vi "Initialize.vi"(7 "Serial Configuration":T1={"Baud Rate"=9600, "Parity"=0, "Data Bits"=8, "Stop Bits"=10, "Flow Control"=0} {"Flow Control" items=["None", "XON/XOFF", "RTS/CTS", "XON/XOFF & RTS/CTS", "DTR/DSR", "XON/XOFF & DTR/DSR"]; "Stop Bits" items=["1.0"=10, "1.5"=15, "2.0"=20]; "Data Bits" items=["7"=7, "8"=8]; "Parity" items=["None", "Odd", "Even", "Mark", "Space"]; "Baud Rate" items=["300"=300, "600"=600, "1200"=1200, "2400"=2400, "4800"=4800, "9600"=9600, "19200"=19200]}, 8 "error in (no error)":errorcluster, 11 "VISA resource name":refnum<visa-resource-name>) -> (0 "error out":errorcluster, 3 "VISA resource name out":refnum<visa-resource-name>)   [LabVIEW 2012, in "SRS_DG535_Lib.lvlib"]
doc: "Establishes communication with the instrument and optionally performs an instrument identification query and/or an instrument reset. It also places the instrument in a default state needed for other instrument driver operations. Therefore, call this VI before calling other instrument driver VIs for this instrument. Generally, you need to call the Initialize VI only once at the beginning of an application."
uses:
  SRS_DG535_Lib.lvlib
panel:
  # "(c) 2007 <Enter Company Name Here>.  ALL RIGHTS RESERVED."
  # "EDIT: Change control description to remove example text for buses not supported."
  # "EDIT: Serial settings must match those on the physical instrument.  Review user's manual to determine the correct Flow Control protocol for the instrument.  \"None\" is the least robust option for this setting, and could lead to unreliable data transmission."
  # "EDIT: If your instrument does not support ID query or Reset, remove the ID Query or Reset control from the front panel and delete the case structure with the ID Query or Reset code from the block diagram."
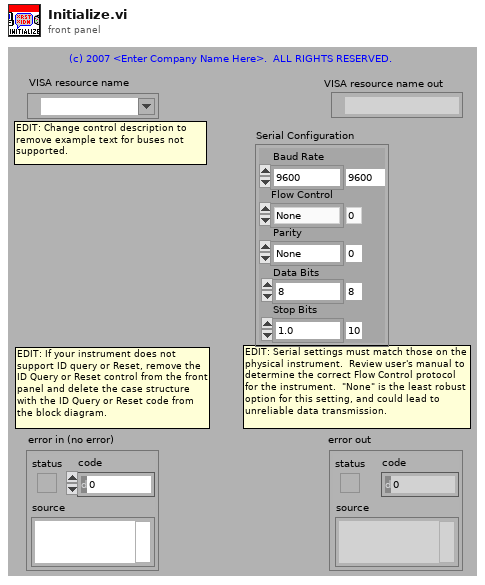
[diagram p1: front panel]
types:
  T1 = cluster{"Baud Rate":u32, "Parity":u16, "Data Bits":u16, "Stop Bits":u16, "Flow Control":u16}
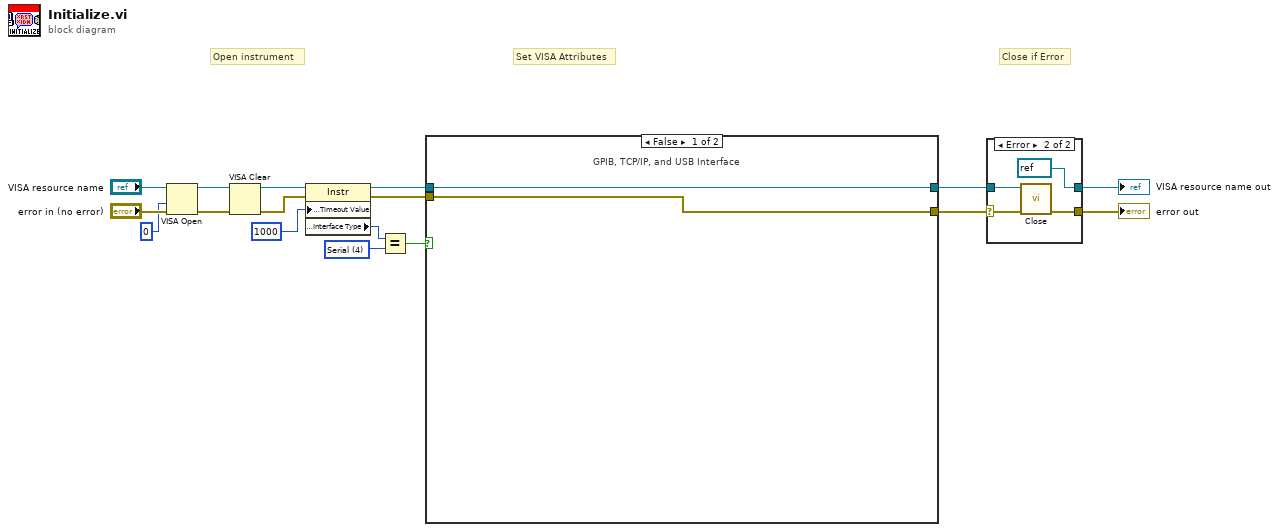
[diagram p0: block diagram]
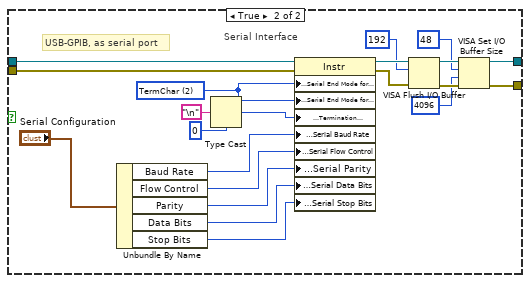
[diagram p2: hidden frame]
diagram:
  w10 = u16 4 items=["GPIB"=1, "VXI"=2, "GPIB-VXI"=3, "Serial"=4, "PXI"=5, "TCPIP"=6, "USB"=7] ("Interface Information:Interface Type")
  # "Set VISA Attributes"
  # "Close if Error"
  # "Open instrument"
  n1 = VISA Open(access mode=u32 0, error in (no error)="error in (no error)", VISA resource name="VISA resource name") -> (VISA resource name=w8:refnum<visa-resource-name>, error out=w7:errorcluster)  [unwired: 2 in]
  n2 = VISA Clear(VISA resource name=w8, error in (no error)=w7) -> (VISA resource name out=w6:refnum<visa-resource-name>, error out=w5:errorcluster)
  n3 = property class="Instr"(reference=w6, error in=w5, "General Settings:Timeout Value"=u32 1000) -> (reference out=w13:refnum<visa-resource-name>, error out=w12:errorcluster, "Interface Information:Interface Type"=w15:u16)
  n4 = Equal?(x=w15, y=w10) -> (x = y?=w11:bool)
  n5 = case shown="False" w11 {
    tunnel: [w18 w37] -> w2
    tunnel: [w19 w34] -> w1
    tunnel: w13 -> [w18 w39]
    tunnel: w12 -> [w19 w40]
    frame False {
      # "GPIB, TCP/IP, and USB Interface"
    }
    frame True {
      w27 = u16 2 items=["None", "LastBit", "TermChar"] ("Serial Settings:Serial End Mode for Reads")
      # "USB-GPIB, as serial port"
      # "Serial Interface"
      n6 = Unbundle By Name("Serial Configuration") -> ("Baud Rate"=w25:u32, "Flow Control"=w21:u16, "Parity"=w23:u16, "Data Bits"=w24:u16, "Stop Bits"=w20:u16)
      n7 = Type Cast(type=u8 0, x="\n") -> (*(type *) &x=w26:u8)
      n8 = property class="Instr"(reference=w39, error in=w40, "Serial Settings:Serial End Mode for Reads"=w27, "Serial Settings:Serial End Mode for Writes"=w27, "Message Based Settings:Termination Character"=w26, "Serial Settings:Serial Baud Rate"=w25, "Serial Settings:Serial Flow Control"=w21, "Serial Settings:Serial Parity"=w23, "Serial Settings:Serial Data Bits"=w24, "Serial Settings:Serial Stop Bits"=w20) -> (reference out=w33:refnum<visa-resource-name>, error out=w36:errorcluster)
      n9 = VISA Flush I/O Buffer(VISA resource name=w33, mask (16)=u16 192, error in (no error)=w36) -> (VISA resource name out=w38:refnum<visa-resource-name>, error out=w35:errorcluster)
      n10 = VISA Set I/O Buffer Size(VISA resource name=w38, mask (16)=u16 48, size (4096)=u32 4096 ("size (0)"), error in (no error)=w35) -> (VISA resource name out=w37:refnum<visa-resource-name>, error out=w34:errorcluster)
    }
  }
  n11 = case shown="Error" w1 {
    selector: w1 -> [w41 w44]
    tunnel: w2 -> [w42 w45]
    tunnel: [w42 refnum<visa-resource-name> refnum ("VISA resource name out")] -> w4
    tunnel: [w41 w46] -> w3
    frame No Error {
    }
    frame Error {
      n12 = call "Close.vi"("error in (no error)"=w44, "VISA resource name"=w45) -> ("error out"=w46:errorcluster)  [unwired: 9 in]
    }
  }
  "VISA resource name out" <- w4
  "error out" <- w3
